vi "BIN_PAQ_FixPath.vi"(6 "path-IN":path, 8 "error in (no error)":errorcluster, 11 "DBAL-BIN in":refnum<class "DBAL-BIN.lvclass">) -> (0 "error out":errorcluster, 3 "DBAL-BIN out":refnum<class "DBAL-BIN.lvclass">, 4 "path-OUT":path)   [LabVIEW 2020, in "Sgraph_lib_V1.lvlib" / "DBAL-BIN.lvclass"]
uses:
  DBAL-BIN.lvclass
  DBAL-BIN.lvclass/DBAL-BIN.ctl
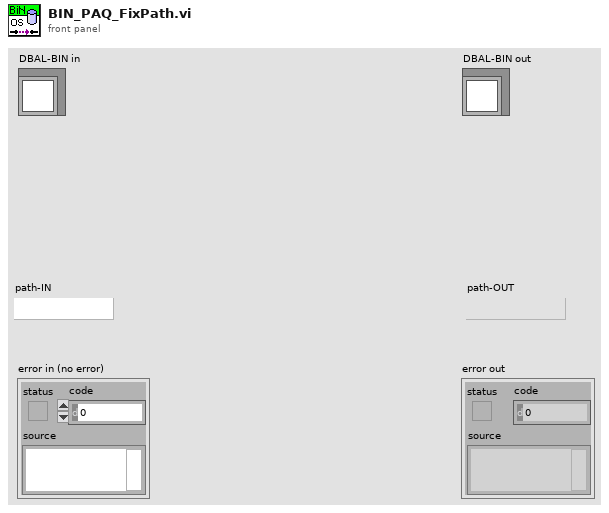
[diagram p1: front panel]
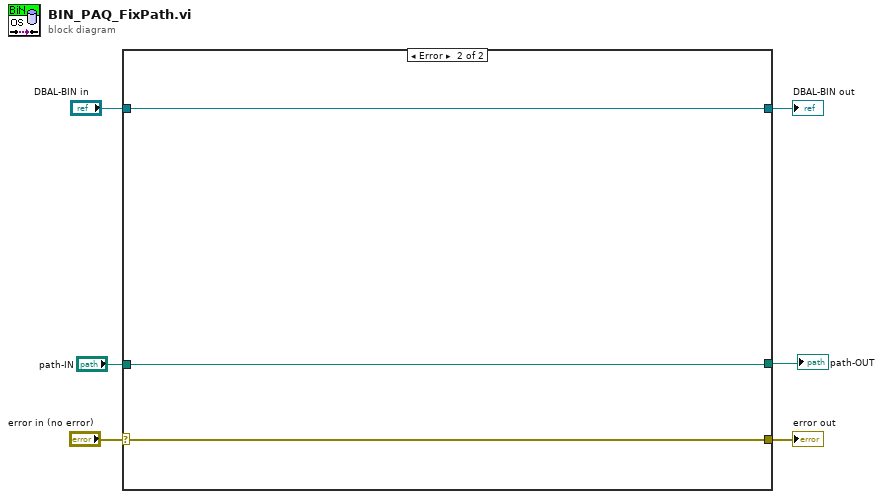
[diagram p0: block diagram]
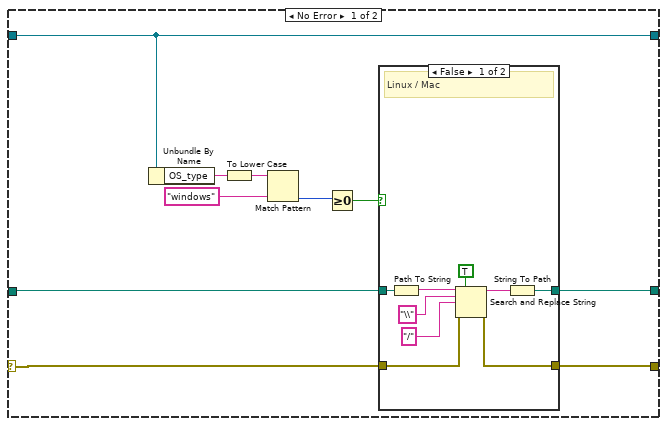
[diagram p2: hidden frame]
diagram:
  n1 = case shown="Error" "error in (no error)" {
    selector: "error in (no error)" -> [w10 w30]
    tunnel: [w9 w30] -> w5
    tunnel: [w11 w29] -> w3
    tunnel: "DBAL-BIN in" -> [w11 w29]
    tunnel: "path-IN" -> [w8 w28]
    tunnel: [w7 w28] -> w1
    frame No Error {
      n2 = Unbundle By Name(w11) -> ("OS_type"=w15:string)
      n3 = To Lower Case(string=w15) -> (all lower case string=w14:string)
      n4 = Match Pattern(string=w14, regular expression="windows") -> (offset past match=w12:i32)  [unwired: 1 in, 3 out]
      n5 = Greater Or Equal To 0?(x=w12) -> (x >= 0?=w16:bool)
      n6 = case shown="False" w16 {
        tunnel: w8 -> [w25 w27]
        tunnel: [w17 w27] -> w7
        tunnel: w10 -> [w20 w26]
        tunnel: [w19 w26] -> w9
        frame False {
          # "Linux / Mac"
          n7 = Path To String(path=w25) -> (string=w24:string)
          n8 = Search and Replace String(replace all?=TRUE ("replace all? (F)"), input string=w24, search string="\\", replace string="/", error in=w20) -> (result string=w18:string, error out=w19:errorcluster)  [unwired: 3 in, 2 out]
          n9 = String To Path(string=w18) -> (path=w17:path)
        }
        frame True {
          # "Windows"
        }
      }
    }
    frame Error {
    }
  }
  "error out" <- w5
  "DBAL-BIN out" <- w3
  "path-OUT" <- w1
